vi "CalculateDelta_t.vi"(10 "InterpFactor":i32, 11 "Array":dbl[](array[numeric])) -> (1 "Reporting Rate":dbl, 3 "delta_t":dbl)   [LabVIEW 2017, in "AppPlugins.lvlib" / "ModelValidationPlugin.lvclass"]
uses:
  ModelValidationPlugin.lvclass
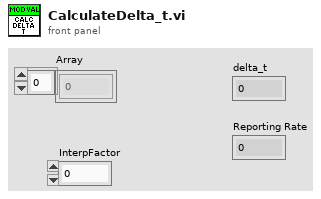
[diagram p1: front panel]
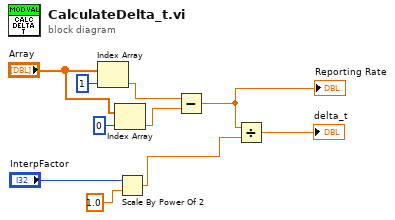
[diagram p0: block diagram]
diagram:
  n1 = Index Array(array="Array", index=1) -> (element=w7:dbl)
  n2 = Index Array(array="Array", index=0) -> (element=w6:dbl)
  n3 = Scale By Power Of 2(n="InterpFactor", x=1.0) -> (x*2^n=w3:dbl)
  n4 = Subtract(x=w7, y=w6) -> (x-y=w1:dbl)
  "Reporting Rate" <- w1
  n5 = Divide(x=w1, y=w3) -> (x/y=→"delta_t":dbl)
